vi "Process Data Time.vi"() -> (2 "Integrated time":dbl, 3 "Loop time":dbl)   [LabVIEW 2019]
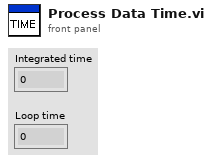
[diagram p1: front panel]
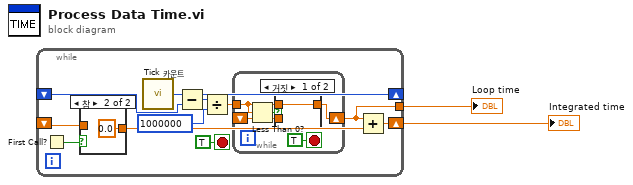
[diagram p0: block diagram]
diagram:
  n1 = while {
    shift-right: [w9] -> _
    shift-left: _ -> [w8]
    shift-right: [w7] -> w2
    shift-left: _ -> [w3]
    tunnel: [w6] -> w1
    stop <- TRUE stop-if-true
    n2 = First Call?() -> (First Call?: T/F=w5:bool)
    n3 = case shown="참" w5 {
      tunnel: [w14 0.0] -> w4
      tunnel: w3 -> [w14 _]
      frame False {
      }
      frame True {
      }
    }
    n4 = call "Tick 카운트"() -> ("Tick Count(uSec)"=w9:u32)
    n5 = Subtract(x=w9, y=w8) -> (x-y=w13:u32)
    n6 = Divide(x=w13, y=u32 1000000) -> (x/y=w11:dbl)
    n7 = while {
      tunnel: w11 -> [w19]
      shift-right: [w18] -> w6
      shift-left: _ -> [w17]
      stop <- TRUE stop-if-true
      n8 = Less Than 0?(x=w19) -> (x < 0?=w20:bool)
      n9 = case shown="거짓" w20 {
        tunnel: [w21 w22] -> w18
        tunnel: w19 -> [w21 _]
        tunnel: w17 -> [_ w22]
        frame False {
        }
        frame True {
        }
      }
    }
    n10 = Add(x=w6, y=w4) -> (x+y=w7:dbl)
  }
  "Integrated time" <- w2
  "Loop time" <- w1
